vi "ActionVIOnCompile.vi"(8 "error in (no error)":errorcluster, 11 "Device Item Ref in":T1 format="%.0x") -> (0 "error out":errorcluster)   [LabVIEW 2020, in "AIM ARINC 664 System Explorer.lvlib"]
uses:
  AIM ARINC 664 System Explorer.lvlib
  <vilib>/NI VeriStand/Custom Device API/Custom Device API.lvlib
  Shared/Compiled.Settings.ctl
  Shared/AIM ARINC 664 Shared.lvlib
  <vilib>/NI VeriStand/Custom Device API/Data Reference.ctl
  <vilib>/NI VeriStand/Custom Device API/Block Data Reference.ctl
  Shared/Inline Execution Unit Compiled Information.ctl
  Shared/Asynchronous Execution Unit Compiled Information.ctl
  Includes/AIM ARINC 664 System Explorer.lvlibp/System Explorer/Implementation/Implementation.lvlib
  Includes/afdx_custom_device Engine.lvlibp/Engine/Interfaces/Execution Unit Factory/Execution Unit Factory.lvclass
  Includes/afdx_custom_device Engine.lvlibp/Engine/Interfaces/Shared Resources Factory/Shared Resources Factory.lvclass
  <vilib>/NI VeriStand/Custom Device API/Set Item Property (Variant).vi
  Includes/afdx_custom_device Engine.lvlibp/Engine/Implementation/Execution Unit Factory/Execution Unit Factory.lvclass
  Includes/afdx_custom_device Engine.lvlibp/Engine/Implementation/Shared Resources Factory/Shared Resources Factory.lvclass
  <vilib>/NI VeriStand/Custom Device API/Custom Device Item Ref.ctl
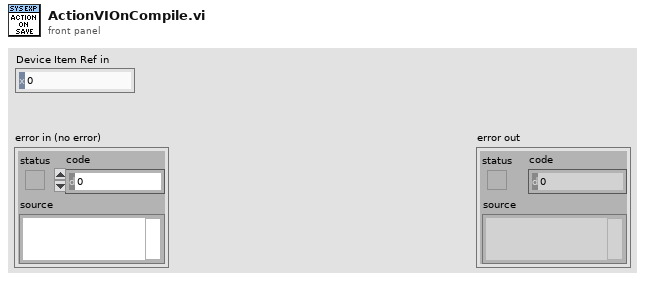
[diagram p1: front panel]
types:
  T1 = typedef "Custom Device API.lvlib/Custom Device Item Ref.ctl" = u64
  T2 = typedef "AIM ARINC 664 System Explorer.lvlibp/Custom Device API.lvlib/Custom Device Item Ref.ctl" = u64
  T3 = typedef "AIM ARINC 664 Shared.lvlib/Compiled.Settings.ctl" = cluster{"Name":string, "Inline Execution Unit Compiled Information":T4[], "Asynchronous Execution Unit Compiled Information":T7[], "Flattened Shared Resources":string}
  T4 = typedef "AIM ARINC 664 Shared.lvlib/Inline Execution Unit Compiled Information.ctl" = cluster{"Flattened Execution Unit":string, "Incoming Buffer":dbl[], "Outgoing Buffer":dbl[], "Incoming Data References":T5[], "Outgoing Data References":T6[]}
  T5 = typedef "Custom Device API.lvlib/Data Reference.ctl" = i32
  T6 = typedef "Custom Device API.lvlib/Block Data Reference.ctl" = cluster{"Data Reference":T5, "Offset":u64, "Length":u64}
  T7 = typedef "AIM ARINC 664 Shared.lvlib/Asynchronous Execution Unit Compiled Information.ctl" = cluster{"Flattened Execution Unit":string, "Incoming Channel Group Name":string, "Outgoing Channel Group Name":string, "ReadWrite Channel Group Name":string}
  T8 = typedef "Custom Device API.lvlib/Custom Device Item Info.ctl" = cluster{"Name":string, "Is Channel":bool, "GUID":string, "Is Waveform":bool}
  T9 = typedef "afdx_custom_device Engine.lvlibp/Interfaces.lvlib/Execution Unit Information.ctl" = cluster{"Execution Unit":refnum<class "Execution Unit.lvclass">, "Incoming Channels":T10[], "Outgoing Channels":T10[], "ReadWrite Channels":T10[]}
  T10 = typedef "afdx_custom_device Engine.lvlibp/Custom Device API.lvlib/Custom Device Item Ref.ctl" = u64
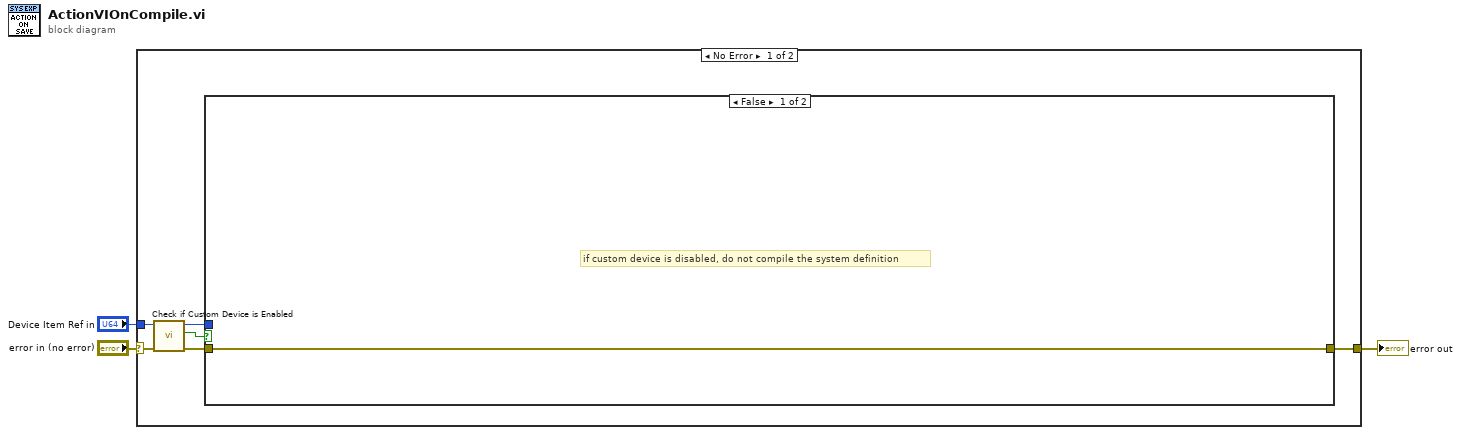
[diagram p0: block diagram]
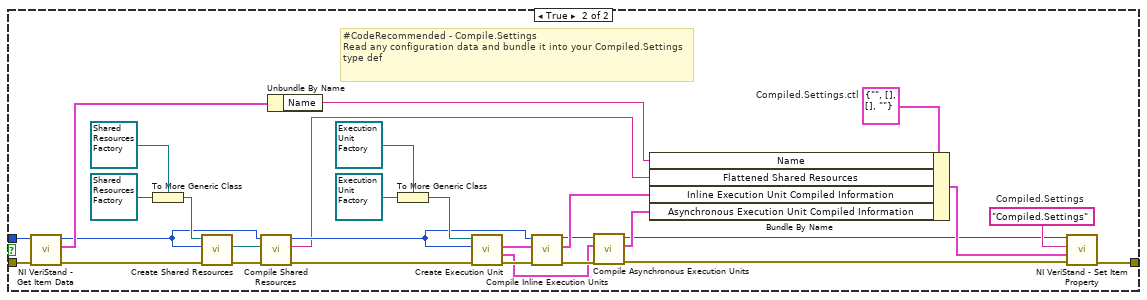
[diagram p2: hidden frame]
diagram:
  n1 = case shown="No Error" "error in (no error)" {
    selector: "error in (no error)" -> [w5 w41]
    tunnel: [w9 w41] -> w2
    tunnel: "Device Item Ref in" -> [w7 _]
    frame No Error {
      n2 = call "Check if Custom Device is Enabled.vi"("error in"=w5, "custom device ref in"=w7) -> ("error out"=w4:errorcluster, "Custom Device is Enabled"=w6:bool, "custom device ref out"=w8:T2)  [unwired: 7 in]
      n3 = case shown="False" w6 {
        tunnel: [w10 w38] -> w9
        tunnel: w4 -> [w10 w35]
        tunnel: w8 -> [_ w33]
        frame False {
          # "if custom device is disabled, do not compile the system definition"
        }
        frame True {
          w36 = T3 {"Name"="", "Inline Execution Unit Compiled Information"=[], "Asynchronous Execution Unit Compiled Information"=[], "Flattened Shared Resources"=""}  # Compiled.Settings.ctl
          w40 = "Compiled.Settings"  # Compiled.Settings
          # "#CodeRecommended - Compile.Settings\nRead any configuration data and bundle it into your Compiled.Settings type def"
          n4 = call <vilib>:"NI VeriStand - Get Item Data.vi"("error in (no error)"=w35, "Item Ref in"=w33) -> ("error out"=w19:errorcluster, "Item Info"=w37:T8, "Item Ref out"=w15:T1)  [unwired: 6 in, 1 out]
          n5 = To More Generic Class(target class=refnum<class "Shared Resources Factory.lvclass"> refnum ("Interfaces.lvlib:Shared Resources Factory.lvclass"), reference=refnum<class "Shared Resources Factory.lvclass"> refnum ("Implementation.lvlib:Shared Resources Factory.lvclass")) -> (generic class reference=w18:refnum<class "Shared Resources Factory.lvclass">)
          n6 = call-dynamic "Create Shared Resources.vi"("error in"=w19, "custom device ref"=w15, "shared resources factory in"=w18) -> ("error out"=w17:errorcluster, "shared resources"=w16:refnum<class "Shared Resources.lvclass">)  [unwired: 6 in, 1 out]
          n7 = call "Compile Shared Resources.vi"("error in"=w17, "shared resources"=w16, "device ref in"=w15) -> ("error out"=w13:errorcluster, "flattened shared resources"=w11:string, "device ref out"=w14:T1)  [unwired: 6 in]
          n8 = Unbundle By Name(w37) -> ("Name"=w12:string)
          n9 = To More Generic Class(target class=refnum<class "Execution Unit Factory.lvclass"> refnum ("Interfaces.lvlib:Execution Unit Factory.lvclass"), reference=refnum<class "Execution Unit Factory.lvclass"> refnum ("Implementation.lvlib:Execution Unit Factory.lvclass")) -> (generic class reference=w32:refnum<class "Execution Unit Factory.lvclass">)
          n10 = call-dynamic "Create Execution Unit.vi"("error in"=w13, "Item Ref"=w14, "Execution Unit Factory in"=w32) -> ("error out"=w34:errorcluster, "Asynchronous Execution Units"=w24:T9[], "Inline Execution Units"=w30:T9[])  [unwired: 5 in, 1 out]
          n11 = call "Compile Inline Execution Units.vi"("error in"=w34, "Inline Execution Units"=w30, "Device Ref in"=w14) -> ("error out"=w29:errorcluster, "Compiled Inline Execution Units"=w31:T4[], "Device Ref out"=w28:T1)  [unwired: 6 in]
          n12 = call "Compile Asynchronous Execution Units.vi"("Device Ref in"=w28, "Asynchronous Execution Units"=w24, "error in"=w29) -> ("Device Ref out"=w25:T1, "Compiled Asynchronous Execution Units"=w27:T7[], "error out"=w26:errorcluster)  [unwired: 5 in]
          n13 = Bundle By Name(cluster=w36, "Name"=w12, "Flattened Shared Resources"=w11, "Inline Execution Unit Compiled Information"=w31, "Asynchronous Execution Unit Compiled Information"=w27) -> (w39:T3)
          n14 = call-poly <vilib>:"NI VeriStand - Set Item Property.vi"("error in (no error)"=w26, "Value"=w39, "Property Name"=w40, "Item Ref in"=w25) -> ("error out"=w38:errorcluster)  [unwired: 5 in, 2 out]
        }
      }
    }
    frame Error {
    }
  }
  "error out" <- w2
